vi "SetupHW.vi"(8 "error in (no error)":errorcluster, 11 "Behavior in":refnum<class "Behavior.lvclass">) -> (0 "error out":errorcluster, 3 "Behavior out":refnum<class "Behavior.lvclass">)   [LabVIEW 2016, in "Behavior.lvclass"]
uses:
  Behavior.lvclass
  Behavior.lvclass/Behavior.ctl
  Cajal - 2016/Photodiode/Photodiode.lvclass
  Cajal - 2016/QuadraturePositionDecoder/QuadraturePositionDecoder.lvclass
  Cajal - 2016/Imaging/Imaging.lvclass
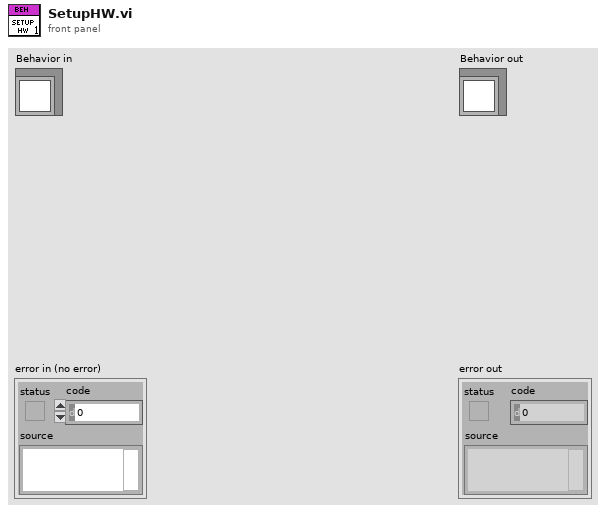
[diagram p1: front panel]
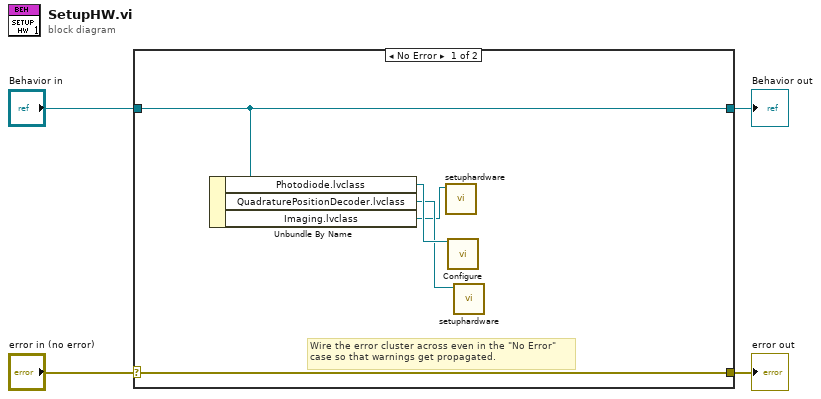
[diagram p0: block diagram]
diagram:
  n1 = case shown="No Error" "error in (no error)" {
    selector: "error in (no error)" -> [w9 w11]
    tunnel: [w9 w11] -> w3
    tunnel: [w8 w10] -> w1
    tunnel: "Behavior in" -> [w8 w10]
    frame No Error {
      # "Wire the error cluster across even in the \"No Error\"\ncase so that warnings get propagated."
      n2 = Unbundle By Name(w8) -> ("Photodiode.lvclass"=w7:refnum<class "Photodiode.lvclass">, "QuadraturePositionDecoder.lvclass"=w6:refnum<class "QuadraturePositionDecoder.lvclass">, "Imaging.lvclass"=w5:refnum<class "Imaging.lvclass">)
      n3 = call-dynamic "setuphardware.vi"("Imaging in"=w5) -> ()  [unwired: 9 in, 2 out]
      n4 = call-dynamic "Configure.vi"("Photodiode in"=w7) -> ()  [unwired: 17 in, 2 out]
      n5 = call-dynamic "setuphardware.vi"("QuadraturePositionDecoder in"=w6) -> ()  [unwired: 9 in, 2 out]
    }
    frame Error {
    }
  }
  "error out" <- w3
  "Behavior out" <- w1
